vi "Should Abort Operation.vi"(8 "New Command Info":T1, 9 "Command Info":T1, 10 "Current Operation":i32, 11 "New Operation":enum16{"Reserve", "Read Current"}(ring)) -> (2 "Execute":bool)   [LabVIEW 2017]
doc: "Determine whether this command will abort the current command before posting it."
uses:
  <vilib>/Rock Robotics/WPI/Framework/Command Status Info.ctl
  <vilib>/Rock Robotics/WPI/Framework/Completion Status.ctl
  <vilib>/Rock Robotics/WPI/Framework/Completion Notifier.ctl
panel:
  # "Determine if the new operation needs to abort.\nHandle the case where we were reserved, perform an action\nand afterwards go back to reserved."
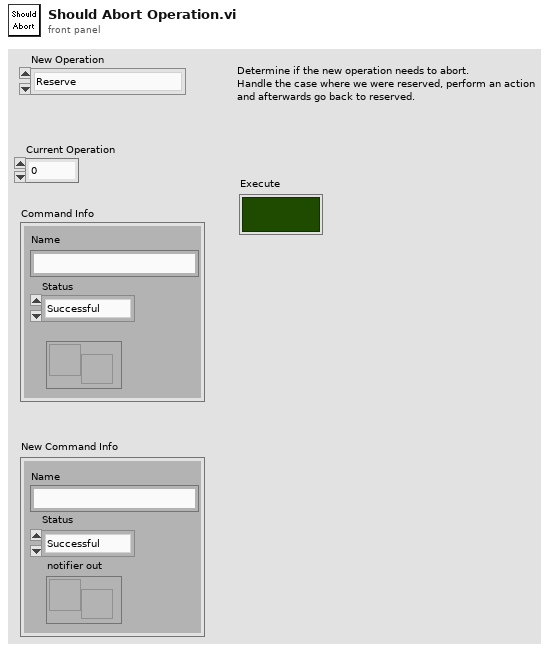
[diagram p1: front panel]
types:
  T1 = typedef "Command Status Info.ctl" = cluster{"Name":string, "Status":T2, "notifier out":T3}
  T2 = typedef "Completion Status.ctl" = enum16{"Successful", "Aborted", "Incomplete"}
  T3 = typedef "Completion Notifier.ctl" = refnum<notifier>
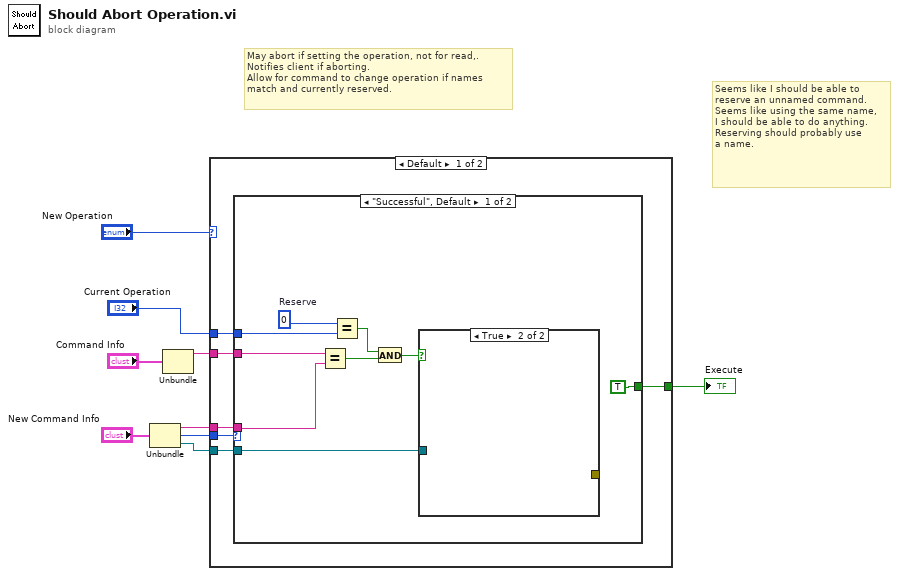
[diagram p0: block diagram]
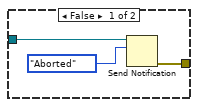
[diagram p2: hidden frame]
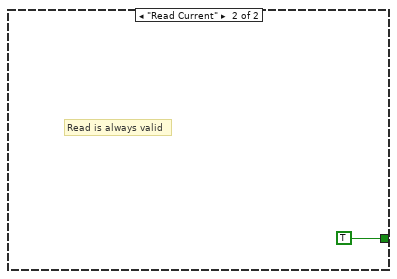
[diagram p4: hidden frame]
diagram:
  # "Seems like I should be able to\nreserve an unnamed command.\nSeems like using the same name,\nI should be able to do anything.\nReserving should probably use\na name."
  # "May abort if setting the operation, not for read,. \nNotifies client if aborting.\nAllow for command to change operation if names\nmatch and currently reserved."
  n1 = Unbundle("New Command Info") -> ("Name"=w6:string, "Status"=w7:T2, "notifier out"=w5:T3)
  n2 = Unbundle("Command Info") -> ("Name"=w3:string)  [unwired: 2 out]
  n3 = case shown="Default" "New Operation" {
    tunnel: w7 -> [w15 _]
    tunnel: w6 -> [w14 _]
    tunnel: w5 -> [w13 _]
    tunnel: [w12 TRUE] -> w4
    tunnel: "Current Operation" -> [w11 _]
    tunnel: w3 -> [w10 _]
    frame Default {
      n4 = case shown="\"Successful\", Default" w15 {
        tunnel: w14 -> [w24 _]
        tunnel: w13 -> [w20 _]
        tunnel: [TRUE _] -> w12
        tunnel: w11 -> [w18 _]
        tunnel: w10 -> [w17 _]
        frame "Successful", Default {
          w16 = 0  # Reserve
          n5 = Equal?(x=w17, y=w24) -> (x = y?=w23:bool)
          n6 = Equal?(x=w16, y=w18) -> (x = y?=w22:bool)
          n7 = And(x=w22, y=w23) -> (x .and. y?=w21:bool)
          n8 = case shown="True" w21 {
            tunnel: w20 -> [w27 _]
            tunnel: [w25 _] -> _
            frame False {
              n9 = Send Notification(notification=Completion_Status."Aborted", notifier=w27) -> (error out=w25:errorcluster)  [unwired: 1 in, 1 out]
            }
            frame True {
            }
          }
        }
        frame "Aborted" {
        }
      }
    }
    frame "Read Current" {
      # "Read is always valid"
    }
  }
  "Execute" <- w4
